vi "sub1.vi"(10 "regular expression":string, 11 "Array":T1(array[cluster])) -> (3 "Tunnel out":refnum<vi>)   [LabVIEW 2020, in "CSM-Helper.lvclass"]
uses:
  CSM-Helper.lvclass
  77a8c2b9-168f-4dc0-b879-7e7d9a594d5e.vi
  77a8c2b9-168f-4dc0-b879-7e7d9a594d5e.vi/eb2405bd-5b2e-436b-9bb3-692ecf4a9268.vi
  77a8c2b9-168f-4dc0-b879-7e7d9a594d5e.vi/c8ad12e3-5e6d-40e1-92e0-1426ef45ec41.vi
  77a8c2b9-168f-4dc0-b879-7e7d9a594d5e.vi/effcbc1a-e97c-42d4-b61f-d821de102707.vi
  CSM-Helper.lvclass/CSM-Helper.ctl
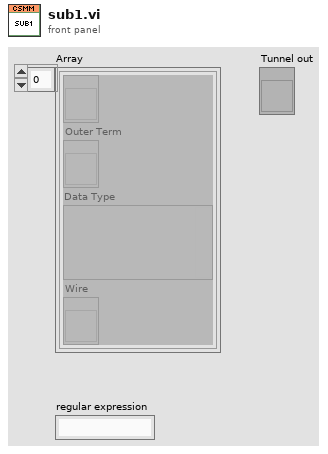
[diagram p1: front panel]
types:
  T1 = cluster{refnum<vi>, "Outer Term":refnum<vi>, "Data Type":variant, "Wire":refnum<vi>}[]
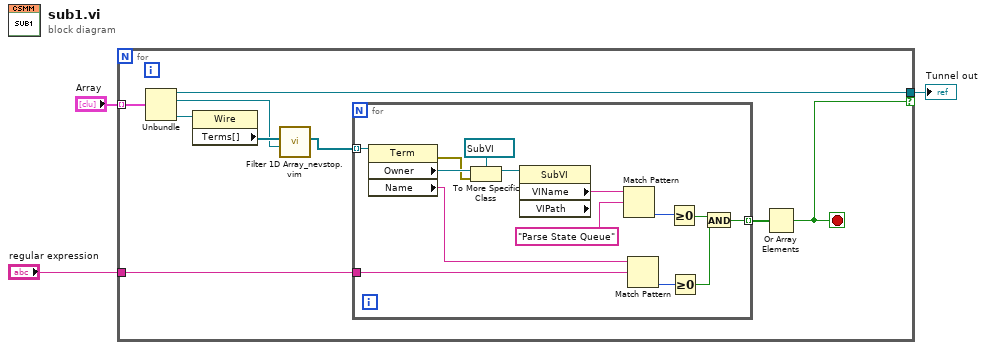
[diagram p0: block diagram]
diagram:
  n1 = for {
    tunnel: "Array" -> [w12] mode=indexing
    tunnel: [w10] -> w2 if=w4
    tunnel: "regular expression" -> [w6]
    stop <- w4 stop-if-true
    n2 = Unbundle(w12) -> (w10:refnum<vi>, "Outer Term"=w8:refnum<vi>, "Wire"=w11:refnum<vi>)  [unwired: 1 out]
    n3 = property class="Wire"(reference=w11) -> ("Terms[]"=w9:refnum<vi>[])  [unwired: 1 in, 2 out]
    n4 = call "Filter 1D Array_nevstop.vim"("items to filter"=w8, "array"=w9) -> ("filtered array"=w5:refnum<vi>[])  [unwired: 4 in, 1 out]
    n5 = for {
      tunnel: [w15] -> w7 mode=indexing
      tunnel: w6 -> [w14]
      tunnel: w5 -> [w13] mode=indexing
      n6 = property class="Term"(reference=w13) -> (error out=w24:errorcluster, "Owner"=w26:refnum<vi>, "Name"=w20:string)  [unwired: 1 in, 1 out]
      n7 = To More Specific Class(target class=refnum<vi> refnum ("Parse State Queue"), reference=w26, error in=w24) -> (specific class reference=w23:refnum<vi>)  [unwired: 1 out]
      n8 = property class="SubVI" props=["VIName", "VIPath"](reference=w23) -> ("VIName"=w22:string)  [unwired: 1 in, 3 out]
      n9 = Match Pattern(string=w22, regular expression="Parse State Queue") -> (offset past match=w19:i32)  [unwired: 1 in, 3 out]
      n10 = Match Pattern(string=w20, regular expression=w14) -> (offset past match=w18:i32)  [unwired: 1 in, 3 out]
      n11 = Greater Or Equal To 0?(x=w19) -> (x >= 0?=w17:bool)
      n12 = Greater Or Equal To 0?(x=w18) -> (x >= 0?=w16:bool)
      n13 = And(x=w17, y=w16) -> (x .and. y?=w15:bool)
    }
    n14 = Or Array Elements(Boolean array=w7) -> (logical OR=w4:bool)
  }
  "Tunnel out" <- w2
